vi "solar_cfg Open.vi"(0 "Config Path (*.ini)":path, 5 "Create File if Necessary (T)":bool=TRUE, 7 "ms Wait for Handle (10000)":i32=10000, 11 "error in (no error)":errorcluster) -> (3 "Filename":string, 4 "Config Refnum":refnum<data-value>, 6 "File Created?":bool, 15 "error out":errorcluster)   [LabVIEW 2018]
doc: "This VI opens a configuration file (*.ini). A semaphore is created to lock access to a configuration file while operations are handled. This VI can handle comments on the same line as the keys. This is able to handle values with or without quotes.\n\n[Section]\nKey = \"Value\" #Comment"
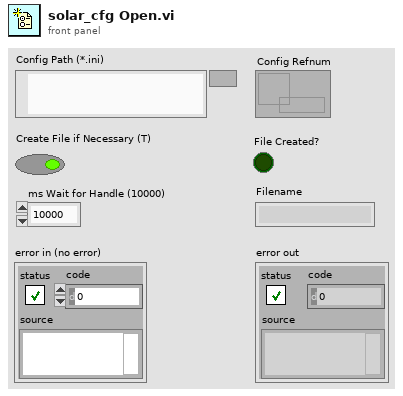
[diagram p1: front panel]
types:
  T1 = enum16{"open", "replace", "create", "open or create", "replace or create", "replace or create with confirmation"}
  T2 = cluster{"Dirty":bool, "Semaphore":refnum<queue>, "Sections":cluster{"Section":string, "kvc":string[][]}[], "Path":path}
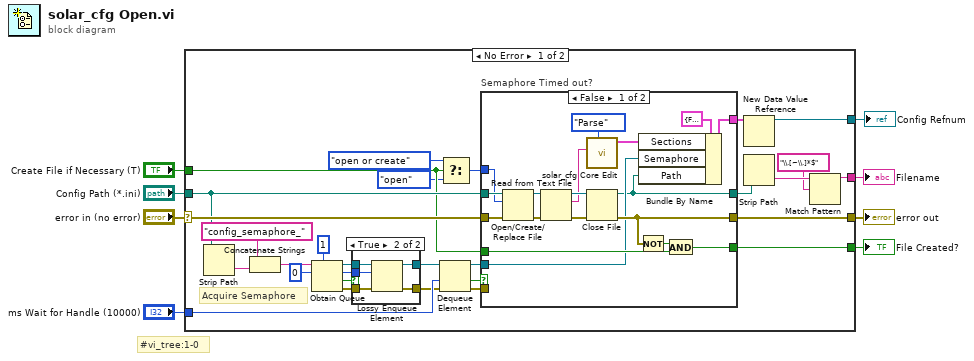
[diagram p0: block diagram]
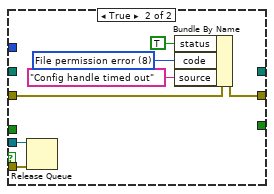
[diagram p3: hidden frame]
diagram:
  # "#vi_tree:1-0"
  n1 = case shown="No Error" "error in (no error)" {
    selector: "error in (no error)" -> [w36 w69]
    tunnel: [w11 w69] -> w7
    tunnel: "Config Path (*.ini)" -> [w35 _]
    tunnel: "ms Wait for Handle (10000)" -> [w34 _]
    tunnel: [w33 _] -> w4
    tunnel: "Create File if Necessary (T)" -> [w32 _]
    tunnel: [w31 _] -> w2
    tunnel: [w9 _] -> w1
    frame No Error {
      w20 = u8 0
      # "Acquire Semaphore"
      n2 = Strip Path(path=w35) -> (name=w27:string)  [unwired: 1 out]
      n3 = Concatenate Strings("config_semaphore_" ("string"), w27) -> (w22:string)
      n4 = Obtain Queue(max queue size (-1, unlimited)=1, name (unnamed)=w22, element data type=w20) -> (queue out=w25:refnum<queue>, created new?=w26:bool, error out=w24:errorcluster)  [unwired: 2 in]
      n5 = case shown="True" w26 {
        tunnel: w25 -> [w38 w43]
        tunnel: w24 -> [w37 w42]
        tunnel: w20 -> [_ w41]
        tunnel: [w38 w40] -> w23
        tunnel: [w37 w39] -> w19
        frame False {
        }
        frame True {
          n6 = Lossy Enqueue Element(queue=w43, element=w41, error in (no error)=w42) -> (queue out=w40:refnum<queue>, error out=w39:errorcluster)  [unwired: 2 out]
        }
      }
      n7 = Dequeue Element(queue=w23, timeout in ms (-1)=w34, error in (no error)=w19) -> (queue out=w17:refnum<queue>, timed out?=w18:bool, error out=w16:errorcluster)  [unwired: 1 out]
      n8 = Select(t=T1."open or create" ("operation (0:open)"), s=w32, f=T1."open" ("operation (0:open)")) -> (s? t:f=w13:T1)
      n9 = case "Semaphore Timed out?" shown="False" w18 {
        tunnel: [w50 w66] -> w11
        tunnel: w36 -> [w56 w65]
        tunnel: w35 -> [w57 _]
        tunnel: w17 -> [w48 w68]
        tunnel: w16 -> [_ w67]
        tunnel: w13 -> [w55 _]
        tunnel: w32 -> [w53 _]
        tunnel: [w52 _] -> w31
        tunnel: [w47 _] -> w12
        tunnel: [w46 _] -> w10
        frame False {
          n10 = Open/Create/Replace File(file path (use dialog)=w57, error in=w56, operation (0:open)=w55) -> (refnum out=w59:refnum<file>, error out=w58:errorcluster)  [unwired: 3 in, 1 out]
          n11 = Read from Text File(file (use dialog)=w59, error in=w58) -> (refnum out=w60:refnum<file>, text=w51:string, error out=w61:errorcluster)  [unwired: 2 in, 1 out]
          n12 = call "solar_cfg Core Edit.vi"("Action (Read)"=enum8{"Read", "Write", "Parse", "Build"}."Parse", "Section/String in"=w51) -> ("Sections out"=w45:cluster{"Section":string, "kvc":string[][]}[])  [unwired: 5 in, 4 out]
          n13 = Close File(refnum=w60, error in=w61) -> (path=w47:path, error out=w50:errorcluster)
          n14 = Not(x=w50) -> (.not. x?=w54:bool)
          n15 = Bundle By Name(cluster=T2 {"Dirty"=FALSE, "Semaphore"=refnum, "Sections"=[], "Path"=path ""} ("Config"), "Sections"=w45, "Semaphore"=w48, "Path"=w47) -> (w46:T2)
          n16 = And(x=w54, y=w53) -> (x .and. y?=w52:bool)
        }
        frame True {
          w64 = u16 8 items=["No error", "Argument error", "Memory is full", "Out of zone", "End of file", "File already open", "Generic file I/O error", "File not found", "File permission error", "Disk is full", "Duplicate path", "Too many files open", "System feature not enabled", "Resource file not found", "Cannot add resource", "Resource not found", "Image not found", "Image memory error", "Pen does not exist", "Config type invalid", "Config token not found", "Config parse error", "Config memory error", "Bad external code format", "Bad external code offset", "External code not present", "Null window", "Destroy window error", "Null menu", "Print aborted", "Bad print record", "Print driver error", "Windows error during printing", "Memory error during printing", "Print dialog error", "Generic print error", "Invalid device refnum", "Device not found", "Device parameter error", "Device unit error", "Cannot open device", "Device call aborted", "Generic error", "Cancelled by user", "Object ID too low", "Object ID too high", "Object not in heap", "Unknown heap", "Unknown object (invalid DefProc)", "Unknown object (DefProc not in table)", "Message out of range", "Invalid (null) method", "Unknown message", "Manager call not supported", "Bad address", "Network operation in progress", "Network operation timed out", "Connection is busy", "Network attribute not supported", "Network error", "Address in use", "System out of memory", "Connection aborted", "Connection refused", "Not connected", "Already connected", "Connection closed", "Initialization error (interapplication manager)", "Bad occurrence", "Wait on unbound occurrence handler", "Occurrence queue overflow", "Datalog type conflict", "Unused", "Unrecognized type (interapplication manager)", "Memory corrupt", "Failed to make temporary DLL", "Old CIN version", "Drag socket not found", "Failed to load drop-object", "Failed to register OLE object", "Failed to release OLE object", "Format specifier type mismatch", "Unknown format specifier", "Too few format specifiers", "Too many format specifiers", "Scan failed", "Newer CIN version", "OLE Convert", "Runtime menu error", "Password tampered", "Unknown error code"]
          n17 = Release Queue(queue=w68, error in (no error)=w67) -> ()  [unwired: 1 in, 3 out]
          n18 = Bundle By Name(cluster=w65, "status"=TRUE, "code"=w64, "source"="Config handle timed out" ("error message (\"\")")) -> (w66:errorcluster)
        }
      }
      n19 = New Data Value Reference(data value=w10) -> (data value reference=w9:refnum<data-value>)  [unwired: 1 in, 1 out]
      n20 = Strip Path(path=w12) -> (name=w30:string)  [unwired: 1 out]
      n21 = Match Pattern(string=w30, regular expression="\\.[~\\.]*$") -> (before substring=w33:string)  [unwired: 4 out]
    }
    frame Error {
    }
  }
  "error out" <- w7
  "Filename" <- w4
  "File Created?" <- w2
  "Config Refnum" <- w1
